vi "Poly_ReadCOMIn.vi"   [LabVIEW 2012]
doc: "Reads the value of the specified COM \"Port\" and returns that value as \"Variable out\"."
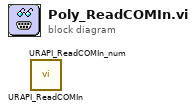
[diagram p0: block diagram]
diagram:
  n1 = call <userlib>:"URAPI_ReadCOMIn.vi"() -> ()  [unwired: 4 in, 2 out]
  n2 = call <userlib>:"URAPI_ReadCOMIn_num.vi"() -> ()  [unwired: 4 in, 2 out]
